vi "USRP_fm_sound_transmitter 2012.vi"() -> ()   [LabVIEW 2012]
doc: "This example shows how simple is to broadcast an Frequency Modulated sound signal using the USRP.\n\n1. Ask the user for a *.wav file.\n2. Read the WAV file.\n3. Select only one channel of the audio data.\n4. Modulate in FM using a frequency deviation of 75kHz. Similar to Radio FM.\n5. Initialize a session.\n6. Configure for arbitrary waveform mode.\n7. Set the output power level and center frequency.\n8. Set the IQ rate to 200k.\n9. Write and read the IQ rate to get the coerced value in order to resample our signal (if needed).\n10. Resample and write the signal to the on board memory. If resample is needed, this step will take little longer depending on the size of the file.\n11. Start the generation.\n12. Check for p the generation.\n13. Stop the generation.\n14. Close the session.\n15. Check for errors."
uses:
  Instance           1 28Saved   fm_sound_transmitter .vi
  <vilib>/sound2/lvsound2.llb/Sound File Info (path).vi
  <vilib>/sound2/lvsound2.llb/Sound File Read Open.vi
  <vilib>/sound2/lvsound2.llb/Sound File Read (DBL).vi
  <vilib>/measure/maresamp.llb/Resample Waveform (continuous).vi
  <instrlib>/niUSRP/niUSRP Write Tx Data (CDB Cluster).vi
  <vilib>/addons/Modulation/niAMT.lvlib
  <vilib>/measure/NI_MAPro.lvlib
panel:
  in  "Digital Gain/Attn":dbl=1.0
  in  "number of samples":i32=-1
  in  "device names":refnum<k15>="192.168.10.2"
  in  "Transmitter Gain":dbl format="%.2f"
  in  "frequency (Hz)":dbl=94700000.0 min=500000.0 max=2700000000.0 format="%.2p"
  out "Status":string="Stopped"
  in  "stop":bool
  out "Audio Data":waveform(dbl)(graph)={"t0"=timestamp(0 s since 1904-01-01), "dt"=9.070294784580499e-05, "Y"=[]}
  # "USRP Configuration"
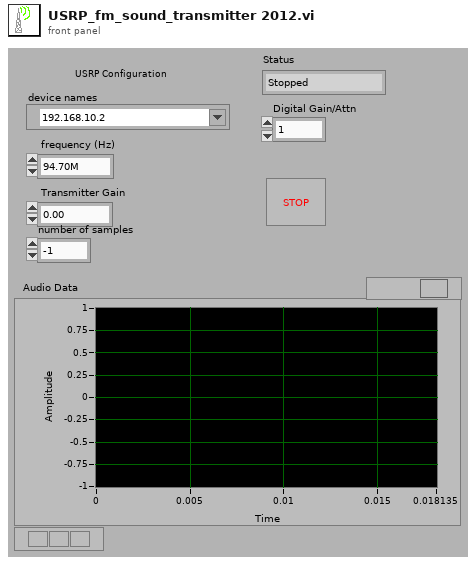
[diagram p1: front panel]
types:
  T1 = typedef "Sound File Refnum.ctl" = refnum<file>
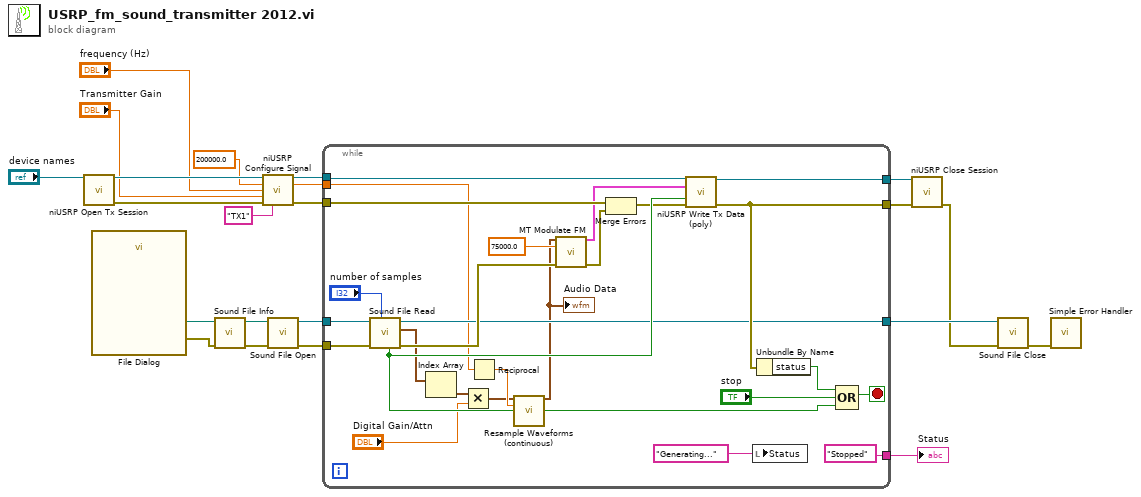
[diagram p0: block diagram]
diagram:
  n1 = call <instrlib>:"niUSRP Open Tx Session.vi"("device names"="device names") -> ("session handle out"=w21:refnum<k15>, "error out"=w20:errorcluster)  [unwired: 13 in]
  n2 = call "File Dialog"() -> ("selected path"=w13:path, "error out"=w8:errorcluster)  [unwired: 12 in, 2 out]
  n3 = call-poly <vilib>:"Sound File Info.vi"("error in (no error)"=w8, "path"=w13) -> ("error out"=w7:errorcluster, "path out"=w9:path)  [unwired: 6 in, 2 out]
  n4 = call <instrlib>:"niUSRP Configure Signal.vi"("session handle"=w21, "IQ rate"=200000.0, "carrier frequency"="frequency (Hz)", "gain"="Transmitter Gain", "error in (no error)"=w20, "active antenna"="TX1") -> ("session handle out"=w15:refnum<k15>, "coerced IQ rate"=w11:dbl, "error out"=w10:errorcluster)  [unwired: 5 in, 2 out]
  n5 = call-poly <vilib>:"Sound File Open.vi"("error in (no error)"=w7, "path"=w9) -> ("error out"=w5:errorcluster, "sound file refnum"=w6:T1)  [unwired: 8 in]
  n6 = while {
    tunnel: ["Stopped" ("Status")] -> w22
    tunnel: w15 -> [w44]
    tunnel: [w43] -> w14
    tunnel: [w42] -> w4
    tunnel: w11 -> [w28]
    tunnel: w10 -> [w31]
    tunnel: w6 -> [w37]
    tunnel: w5 -> [w36]
    tunnel: [w35] -> w3
    stop <- w46 stop-if-true
    n7 = call-poly <vilib>:"Sound File Read.vi"("number of samples/ch (-1: all)"="number of samples", "error in (no error)"=w36, "sound file refnum"=w37) -> ("error out"=w39:errorcluster, "data"=w33:waveform(dbl)[], "sound file refnum out"=w35:T1, "end of file?"=w38:bool)  [unwired: 4 in, 1 out]
    n8 = Index Array(array=w33) -> (element=w25:waveform(dbl))  [unwired: 1 in]
    n9 = Multiply(x=w25, y="Digital Gain/Attn") -> (x*y=w24:waveform(dbl))
    n10 = Reciprocal(x=w28) -> (1/x=w29:dbl)
    n11 = call-poly <vilib>:"Resample Waveforms (continuous).vi"("waveform in"=w24, "dt"=w29) -> ("resampled waveform out"=w26:waveform(dbl))  [unwired: 9 in, 4 out]
    "Audio Data" <- w26
    n12 = call <vilib>:"MT Modulate FM.vi"("message signal"=w26, "FM deviation (Hz)"=75000.0, "error in (no error)"=w39) -> ("FM modulated waveform"=w30:cluster{"t0":dbl, "dt":dbl, "Y":cdb[]}, "error out"=w27:errorcluster)  [unwired: 11 in]
    n13 = Merge Errors(w31, w27) -> (w32:errorcluster)
    n14 = call-poly <instrlib>:"niUSRP Write Tx Data (poly).vi"("session handle"=w44, "data"=w30, "end of data?"=w38, "error in (no error)"=w32) -> ("session handle out"=w43:refnum<k15>, "error out"=w42:errorcluster)  [unwired: 10 in]
    n15 = local write "Status"("Generating..." ("Status")) -> ()
    n16 = Unbundle By Name(w42) -> ("status"=w41:bool)
    n17 = Compound Arithmetic op=OR(w41, "stop", w38) -> (w46:bool)
  }
  "Status" <- w22
  n18 = call <instrlib>:"niUSRP Close Session.vi"("session handle"=w14, "error in (no error)"=w4) -> ("error out"=w1:errorcluster)  [unwired: 13 in]
  n19 = call <vilib>:"Sound File Close.vi"("error in (no error)"=w1, "sound file refnum"=w3) -> ("error out"=w2:errorcluster)  [unwired: 9 in]
  n20 = call <vilib>:"Simple Error Handler.vi"("error in (no error)"=w2) -> ()  [unwired: 4 in, 5 out]
